vi "P541_Init.vi"() -> (1 "Status":bool, 2 "Positions":dbl[](array[numeric]), 3 "VISA Refnum out":refnum<visa-resource-name>)   [LabVIEW 2011]
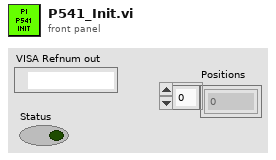
[diagram p1: front panel]
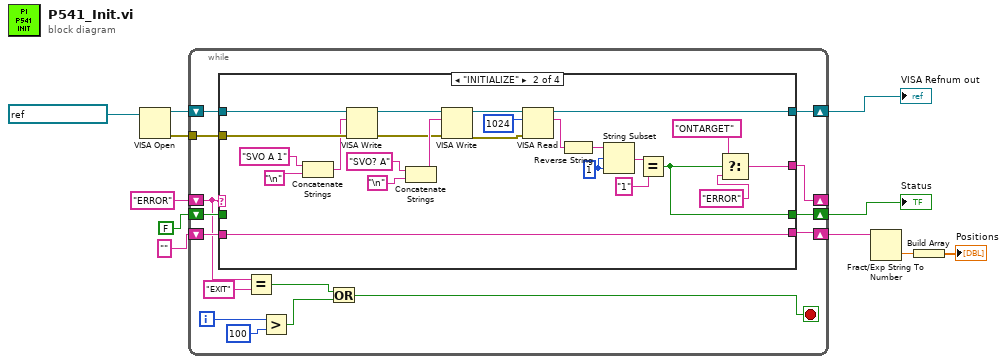
[diagram p0: block diagram]
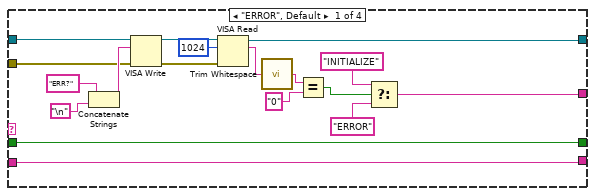
[diagram p2: hidden frame]
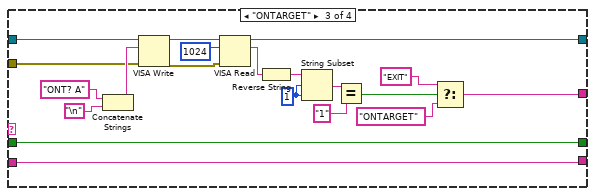
[diagram p3: hidden frame]
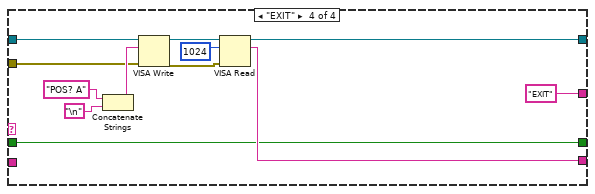
[diagram p4: hidden frame]
diagram:
  n1 = VISA Open(VISA resource name=refnum<visa-resource-name> "PIchassisE816") -> (VISA resource name=w10:refnum<visa-resource-name>, error out=w9:errorcluster)  [unwired: 4 in]
  n2 = while {
    tunnel: w9 -> [w24]
    shift-right: [w23] -> _
    shift-left: "ERROR" ("string") -> [w15]
    shift-right: [w26] -> w11
    shift-left: FALSE -> [w20]
    shift-right: [w21] -> w3
    shift-left: "" ("read buffer") -> [w19]
    shift-right: [w22] -> w6
    shift-left: w10 -> [w25]
    i -> [w18]
    stop <- w13 stop-if-true
    n3 = case shown="\"INITIALIZE\"" w15 {
      tunnel: [w27 w47 w70 w89] -> w26
      tunnel: w25 -> [w40 w68 w73 w94]
      tunnel: w24 -> [w38 w66 w72 w93]
      tunnel: [w30 w50 w77 "EXIT" ("string")] -> w23
      tunnel: [w29 w45 w71 w90] -> w22
      tunnel: [w28 w46 w69 w91] -> w21
      tunnel: w20 -> [w27 _ w70 w89]
      tunnel: w19 -> [w28 w46 w69 _]
      frame "ERROR", Default {
        n4 = Concatenate Strings("ERR?" ("string"), "\n") -> (w43:string)
        n5 = VISA Write(VISA resource name=w40, write buffer=w43, error in (no error)=w38) -> (VISA resource name out=w44:refnum<visa-resource-name>, error out=w37:errorcluster)  [unwired: 1 out]
        n6 = VISA Read(VISA resource name=w44, byte count=u32 1024, error in (no error)=w37) -> (VISA resource name out=w29:refnum<visa-resource-name>, read buffer=w36:string)  [unwired: 2 out]
        n7 = call <vilib>:"Trim Whitespace.vi"("string"=w36) -> ("trimmed string"=w34:string)  [unwired: 1 in]
        n8 = Equal?(x=w34, y="0") -> (x = y?=w33:bool)
        n9 = Select(t="INITIALIZE", s=w33, f="ERROR" ("string")) -> (s? t:f=w30:string)
      }
      frame "INITIALIZE" {
        w61 = 1 ("length (rest)")
        n10 = Concatenate Strings("SVO A 1" ("string"), "\n") -> (w51:string)
        n11 = VISA Write(VISA resource name=w68, write buffer=w51, error in (no error)=w66) -> (VISA resource name out=w55:refnum<visa-resource-name>, error out=w54:errorcluster)  [unwired: 1 out]
        n12 = Concatenate Strings("SVO? A" ("string"), "\n") -> (w64:string)
        n13 = VISA Write(VISA resource name=w55, write buffer=w64, error in (no error)=w54) -> (VISA resource name out=w57:refnum<visa-resource-name>, error out=w56:errorcluster)  [unwired: 1 out]
        n14 = VISA Read(VISA resource name=w57, byte count=u32 1024, error in (no error)=w56) -> (VISA resource name out=w45:refnum<visa-resource-name>, read buffer=w60:string)  [unwired: 2 out]
        n15 = Reverse String(1:w60) -> (0:w62:string)
        n16 = String Subset(string=w62, offset (0)=w61, length (rest)=w61) -> (substring=w59:string)
        n17 = Equal?(x=w59, y="1") -> (x = y?=w47:bool)
        n18 = Select(t="ONTARGET" ("string"), s=w47, f="ERROR" ("string")) -> (s? t:f=w50:string)
      }
      frame "ONTARGET" {
        w83 = 1 ("length (rest)")
        n19 = Concatenate Strings("ONT? A" ("string"), "\n") -> (w86:string)
        n20 = VISA Write(VISA resource name=w73, write buffer=w86, error in (no error)=w72) -> (VISA resource name out=w79:refnum<visa-resource-name>, error out=w78:errorcluster)  [unwired: 1 out]
        n21 = VISA Read(VISA resource name=w79, byte count=u32 1024, error in (no error)=w78) -> (VISA resource name out=w71:refnum<visa-resource-name>, read buffer=w82:string)  [unwired: 2 out]
        n22 = Reverse String(1:w82) -> (0:w84:string)
        n23 = String Subset(string=w84, offset (0)=w83, length (rest)=w83) -> (substring=w81:string)
        n24 = Equal?(x=w81, y="1") -> (x = y?=w74:bool)
        n25 = Select(t="EXIT" ("string"), s=w74, f="ONTARGET" ("string")) -> (s? t:f=w77:string)
      }
      frame "EXIT" {
        n26 = Concatenate Strings("POS? A" ("string"), "\n") -> (w98:string)
        n27 = VISA Write(VISA resource name=w94, write buffer=w98, error in (no error)=w93) -> (VISA resource name out=w96:refnum<visa-resource-name>, error out=w95:errorcluster)  [unwired: 1 out]
        n28 = VISA Read(VISA resource name=w96, byte count=u32 1024, error in (no error)=w95) -> (VISA resource name out=w90:refnum<visa-resource-name>, read buffer=w91:string)  [unwired: 2 out]
      }
    }
    n29 = Equal?(x=w15, y="EXIT") -> (x = y?=w14:bool)
    n30 = Greater?(x=w18, y=100 ("x")) -> (0:w16:bool)
    n31 = Or(x=w14, y=w16) -> (x .or. y?=w13:bool)
  }
  "Status" <- w11
  "VISA Refnum out" <- w6
  n32 = Fract/Exp String To Number(string=w3) -> (number=w2:dbl)  [unwired: 3 in, 1 out]
  n33 = Build Array(w2) -> (→"Positions":dbl[])
